vi "FlatToRichnidaqmx_grpc_ReadCounterScalarF64Request.vi"(5 "OutputClusterType":T1, 11 "InputCluster":T3) -> (3 "OutputCluster":T1)   [LabVIEW 2021, in "NI DAQmx_server.lvlib"]
uses:
  NI DAQmx_server.lvlib
  nidaqmx_grpc_ReadCounterScalarF64Request_Flat.ctl
  nidevice_grpc_Session_Flat.ctl
  nidaqmx_grpc_ReadCounterScalarF64Request.ctl
  nidevice_grpc_Session_session/nidevice_grpc_Session_session.lvclass
  nidevice_grpc_Session.ctl
  nidevice_grpc_Session_session/nidevice_grpc_Session_session.lvclass/nidevice_grpc_Session_session.ctl
  nidevice_grpc_Session_session/Setname.vi
  nidevice_grpc_Session_session/Setid.vi
  nidevice_grpc_Session_session/GetFieldFromProtobufIndexnidevice_grpc_Session_session.vi
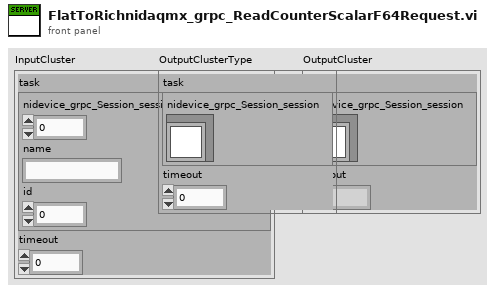
[diagram p1: front panel]
types:
  T1 = typedef "NI DAQmx_server.lvlib/nidaqmx_grpc_ReadCounterScalarF64Request.ctl" = cluster{"task":T2, "timeout":dbl}
  T2 = typedef "NI DAQmx_server.lvlib/nidevice_grpc_Session.ctl" = cluster{"nidevice_grpc_Session_session":refnum<class "nidevice_grpc_Session_session.lvclass">}
  T3 = typedef "NI DAQmx_server.lvlib/nidaqmx_grpc_ReadCounterScalarF64Request_Flat.ctl" = cluster{"task":T4, "timeout":dbl}
  T4 = typedef "NI DAQmx_server.lvlib/nidevice_grpc_Session_Flat.ctl" = cluster{"nidevice_grpc_Session_session_selected_index":i32, "name":string, "id":u32}
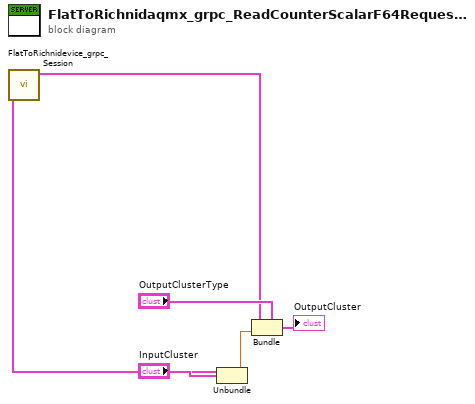
[diagram p0: block diagram]
diagram:
  n1 = Unbundle "Unbundle"("InputCluster") -> ("task"=w3:T4, "timeout"=w1:dbl)
  n2 = call "FlatToRichnidevice_grpc_Session.vi"("InputCluster"=w3) -> ("OutputCluster"=w2:T2)  [unwired: 10 in]
  n3 = Bundle "Bundle"(cluster="OutputClusterType", "task"=w2, "timeout"=w1) -> (→"OutputCluster":T1)
